vi "_old_Load_SetList_Convert_v2.2_to_v4.vi"(0 "Path":path=path "G:/experiment/Data Acquisition/Hardware Control/procedures/23July07_Evaporate_AO_NoRF_NiceBEC_XY_Opt_Abigail", 1 "error in (no error)":errorcluster) -> (2 "Procedure Name":string="IBS_PICameraTest_29Sep04", 3 "Paramaters":T1={"Master PB Staging List"=[{"Output Bits"=[], "Delay (s)"="", "String"="", "Halt?"=FALSE}, {"Output Bits"=[], "Delay (s)"="", "String"="", "Halt?"=FALSE}, {"Output Bits"=[], "Delay (s)"="", "String"="", "Halt?"=FALSE}, {"Output Bits"=[], "Delay (s)"="", "String"="", "Halt?"=FALSE}, {"Output Bits"=[], "Delay (s)"="", "String"="", "Halt?"=FALSE}, {"Output Bits"=[], "Delay (s)"="", "String"="", "Halt?"=FALSE}, {"Output Bits"=[], "Delay (s)"="", "String"="", "Halt?"=FALSE}, {"Output Bits"=[], "Delay (s)"="", "String"="", "Halt?"=FALSE}, {"Output Bits"=[], "Delay (s)"="", "String"="", "Halt?"=FALSE}, {"Output Bits"=[], "Delay (s)"="", "String"="", "Halt?"=FALSE}, {"Output Bits"=[], "Delay (s)"="", "String"="", "Halt?"=FALSE}, {"Output Bits"=[], "Delay (s)"="", "String"="", "Halt?"=FALSE}, {"Output Bits"=[], "Delay (s)"="", "String"="", "Halt?"=FALSE}, {"Output Bits"=[], "Delay (s)"="", "String"="", "Halt?"=FALSE}, {"Output Bits"=[], "Delay (s)"="", "String"="", "Halt?"=FALSE}, {"Output Bits"=[], "Delay (s)"="", "String"="", "Halt?"=FALSE}, {"Output Bits"=[], "Delay (s)"="", "String"="", "Halt?"=FALSE}, {"Output Bits"=[], "Delay (s)"="", "String"="", "Halt?"=FALSE}, {"Output Bits"=[], "Delay (s)"="", "String"="", "Halt?"=FALSE}, {"Output Bits"=[], "Delay (s)"="", "String"="", "Halt?"=FALSE}, {"Output Bits"=[], "Delay (s)"="", "String"="", "Halt?"=FALSE}, {"Output Bits"=[], "Delay (s)"="", "String"="", "Halt?"=FALSE}, {"Output Bits"=[], "Delay (s)"="", "String"="", "Halt?"=FALSE}, {"Output Bits"=[], "Delay (s)"="", "String"="", "Halt?"=FALSE}, {"Output Bits"=[], "Delay (s)"="", "String"="", "Halt?"=FALSE}, {"Output Bits"=[], "Delay (s)"="", "String"="", "Halt?"=FALSE}, {"Output Bits"=[], "Delay (s)"="", "String"="", "Halt?"=FALSE}, {"Output Bits"=[], "Delay (s)"="", "String"="", "Halt?"=FALSE}, {"Output Bits"=[], "Delay (s)"="", "String"="", "Halt?"=FALSE}, {"Output Bits"=[], "Delay (s)"="", "String"="", "Halt?"=FALSE}, {"Output Bits"=[], "Delay (s)"="", "String"="", "Halt?"=FALSE}, {"Output Bits"=[], "Delay (s)"="", "String"="", "Halt?"=FALSE}, {"Output Bits"=[], "Delay (s)"="", "String"="", "Halt?"=FALSE}, {"Output Bits"=[], "Delay (s)"="", "String"="", "Halt?"=FALSE}, {"Output Bits"=[], "Delay (s)"="", "String"="", "Halt?"=FALSE}, {"Output Bits"=[], "Delay (s)"="", "String"="", "Halt?"=FALSE}, {"Output Bits"=[], "Delay (s)"="", "String"="", "Halt?"=FALSE}, {"Output Bits"=[], "Delay (s)"="", "String"="", "Halt?"=FALSE}, {"Output Bits"=[], "Delay (s)"="", "String"="", "Halt?"=FALSE}, {"Output Bits"=[], "Delay (s)"="", "String"="", "Halt?"=FALSE}, {"Output Bits"=[], "Delay (s)"="", "String"="", "Halt?"=FALSE}, {"Output Bits"=[], "Delay (s)"="", "String"="", "Halt?"=FALSE}, {"Output Bits"=[], "Delay (s)"="", "String"="", "Halt?"=FALSE}, {"Output Bits"=[], "Delay (s)"="", "String"="", "Halt?"=FALSE}], "Slave PB Staging List"=[{"Output Bits"=[], "Delay (s)"="", "String"="", "Halt?"=FALSE}, {"Output Bits"=[], "Delay (s)"="", "String"="", "Halt?"=FALSE}, {"Output Bits"=[], "Delay (s)"="", "String"="", "Halt?"=FALSE}, {"Output Bits"=[], "Delay (s)"="", "String"="", "Halt?"=FALSE}, {"Output Bits"=[], "Delay (s)"="", "String"="", "Halt?"=FALSE}, {"Output Bits"=[], "Delay (s)"="", "String"="", "Halt?"=FALSE}, {"Output Bits"=[], "Delay (s)"="", "String"="", "Halt?"=FALSE}, {"Output Bits"=[], "Delay (s)"="", "String"="", "Halt?"=FALSE}, {"Output Bits"=[], "Delay (s)"="", "String"="", "Halt?"=FALSE}, {"Output Bits"=[], "Delay (s)"="", "String"="", "Halt?"=FALSE}, {"Output Bits"=[], "Delay (s)"="", "String"="", "Halt?"=FALSE}, {"Output Bits"=[], "Delay (s)"="", "String"="", "Halt?"=FALSE}, {"Output Bits"=[], "Delay (s)"="", "String"="", "Halt?"=FALSE}, {"Output Bits"=[], "Delay (s)"="", "String"="", "Halt?"=FALSE}, {"Output Bits"=[], "Delay (s)"="", "String"="", "Halt?"=FALSE}, {"Output Bits"=[], "Delay (s)"="", "String"="", "Halt?"=FALSE}, {"Output Bits"=[], "Delay (s)"="", "String"="", "Halt?"=FALSE}, {"Output Bits"=[], "Delay (s)"="", "String"="", "Halt?"=FALSE}, {"Output Bits"=[], "Delay (s)"="", "String"="", "Halt?"=FALSE}, {"Output Bits"=[], "Delay (s)"="", "String"="", "Halt?"=FALSE}, {"Output Bits"=[], "Delay (s)"="", "String"="", "Halt?"=FALSE}, {"Output Bits"=[], "Delay (s)"="", "String"="", "Halt?"=FALSE}, {"Output Bits"=[], "Delay (s)"="", "String"="", "Halt?"=FALSE}, {"Output Bits"=[], "Delay (s)"="", "String"="", "Halt?"=FALSE}, {"Output Bits"=[], "Delay (s)"="", "String"="", "Halt?"=FALSE}, {"Output Bits"=[], "Delay (s)"="", "String"="", "Halt?"=FALSE}, {"Output Bits"=[], "Delay (s)"="", "String"="", "Halt?"=FALSE}, {"Output Bits"=[], "Delay (s)"="", "String"="", "Halt?"=FALSE}, {"Output Bits"=[], "Delay (s)"="", "String"="", "Halt?"=FALSE}, {"Output Bits"=[], "Delay (s)"="", "String"="", "Halt?"=FALSE}, {"Output Bits"=[], "Delay (s)"="", "String"="", "Halt?"=FALSE}, {"Output Bits"=[], "Delay (s)"="", "String"="", "Halt?"=FALSE}, {"Output Bits"=[], "Delay (s)"="", "String"="", "Halt?"=FALSE}, {"Output Bits"=[], "Delay (s)"="", "String"="", "Halt?"=FALSE}, {"Output Bits"=[], "Delay (s)"="", "String"="", "Halt?"=FALSE}, {"Output Bits"=[], "Delay (s)"="", "String"="", "Halt?"=FALSE}, {"Output Bits"=[], "Delay (s)"="", "String"="", "Halt?"=FALSE}, {"Output Bits"=[], "Delay (s)"="", "String"="", "Halt?"=FALSE}, {"Output Bits"=[], "Delay (s)"="", "String"="", "Halt?"=FALSE}, {"Output Bits"=[], "Delay (s)"="", "String"="", "Halt?"=FALSE}, {"Output Bits"=[], "Delay (s)"="", "String"="", "Halt?"=FALSE}, {"Output Bits"=[], "Delay (s)"="", "String"="", "Halt?"=FALSE}, {"Output Bits"=[], "Delay (s)"="", "String"="", "Halt?"=FALSE}, {"Output Bits"=[], "Delay (s)"="", "String"="", "Halt?"=FALSE}], "Novatech Ramps"=[{"Ramp Channels"=[], "2 Freq. [MHz]"="", "2 Power [dBm]"="", "3 Freq. [MHz]"="", "3 Power [dBm]"="", "Serial Port"=""}, {"Ramp Channels"=[], "2 Freq. [MHz]"="", "2 Power [dBm]"="", "3 Freq. [MHz]"="", "3 Power [dBm]"="", "Serial Port"=""}, {"Ramp Channels"=[], "2 Freq. [MHz]"="", "2 Power [dBm]"="", "3 Freq. [MHz]"="", "3 Power [dBm]"="", "Serial Port"=""}, {"Ramp Channels"=[], "2 Freq. [MHz]"="", "2 Power [dBm]"="", "3 Freq. [MHz]"="", "3 Power [dBm]"="", "Serial Port"=""}, {"Ramp Channels"=[], "2 Freq. [MHz]"="", "2 Power [dBm]"="", "3 Freq. [MHz]"="", "3 Power [dBm]"="", "Serial Port"=""}, {"Ramp Channels"=[], "2 Freq. [MHz]"="", "2 Power [dBm]"="", "3 Freq. [MHz]"="", "3 Power [dBm]"="", "Serial Port"=""}, {"Ramp Channels"=[], "2 Freq. [MHz]"="", "2 Power [dBm]"="", "3 Freq. [MHz]"="", "3 Power [dBm]"="", "Serial Port"=""}], "Sequencing Info"=[{"Start"=0.0, "End"=2.11, "Sequenced Data"=[], "Inform\nIgor?"=FALSE, "Computed Step Size"=0.0, "Procedure Variable"="", "Default"=2.11, "Steps"=0}], "SRS Ramps"=[{"lattice ramp"=[{"dt"="", "formula"=""}, {"dt"="", "formula"=""}, {"dt"="", "formula"=""}], "Output"=[{"Time Values"=[0.0, 0.002, 0.004, 0.006, 0.008, 0.01, 0.012, 0.014, 0.016, 0.018000000000000002, 0.02, 0.022, 0.024, 0.026000000000000002, 0.028, 0.03, 0.032, 0.034, 0.036000000000000004, 0.038, 0.04, 0.042, 0.044, 0.046, 0.048, 0.05, 0.052000000000000005, 0.054, 0.056, 0.058, 0.06, 0.062, 0.064, 0.066, 0.068, 0.07, 0.07200000000000001, 0.074, 0.076, 0.078, 0.08, 0.082, 0.084, 0.08600000000000001, 0.088, 0.09, 0.092, 0.094, 0.096, 0.098, 0.1, 0.10200000000000001, 0.10400000000000001, 0.106, 0.108, 0.11, 0.112, 0.114, 0.116, 0.11800000000000001, 0.12, 0.122, 0.124, 0.126, 0.128, 0.13, 0.132, 0.134, 0.136, 0.138, 0.14, 0.14200000000000002, 0.14400000000000002, 0.146, 0.148, 0.15, 0.152, 0.154, 0.156, 0.158, 0.16, 0.162, 0.164, 0.166, 0.168, 0.17, 0.17200000000000001, 0.17400000000000002, 0.176, 0.178, 0.18, 0.182, 0.184, 0.186, 0.188, 0.19, 0.192, 0.194, 0.196, 0.198, 0.2, 0.6000000000000001, 0.6000000000000001, 0.6002000000000001, 0.6004, 0.6006000000000001, 0.6008000000000001, 0.6010000000000001, 0.6012000000000001, 0.6014, 0.6016000000000001, 0.6018000000000001, 0.6020000000000001, 0.6022000000000001, 0.6024, 0.6026000000000001, 0.6028000000000001, 0.6030000000000001, 0.6032000000000001, 0.6034, 0.6036000000000001, 0.6038000000000001, 0.6040000000000001, 0.6042000000000001, 0.6044, 0.6046000000000001, 0.6048000000000001, 0.6050000000000001, 0.6052000000000001, 0.6054, 0.6056000000000001, 0.6058000000000001, 0.6060000000000001, 0.6062000000000001, 0.6064, 0.6066000000000001, 0.6068000000000001, 0.6070000000000001, 0.6072000000000001, 0.6074, 0.6076000000000001, 0.6078000000000001, 0.6080000000000001, 0.6082000000000001, 0.6084, 0.6086000000000001, 0.6088000000000001, 0.6090000000000001, 0.6092000000000001, 0.6094, 0.6096000000000001, 0.6098000000000001, 0.6100000000000001, 0.6102000000000001, 0.6104, 0.6106000000000001, 0.6108000000000001, 0.6110000000000001, 0.6112000000000001, 0.6114, 0.6116000000000001, 0.6118000000000001, 0.6120000000000001, 0.6122000000000001, 0.6124, 0.6126, 0.6128000000000001, 0.6130000000000001, 0.6132000000000001, 0.6134000000000001, 0.6136000000000001, 0.6138000000000001, 0.6140000000000001, 0.6142000000000001, 0.6144000000000001, 0.6146, 0.6148000000000001, 0.6150000000000001, 0.6152000000000001, 0.6154000000000001, 0.6156, 0.6158000000000001, 0.6160000000000001, 0.6162000000000001, 0.6164000000000001, 0.6166, 0.6168000000000001, 0.6170000000000001, 0.6172000000000001, 0.6174000000000001, 0.6176, 0.6178000000000001, 0.6180000000000001, 0.6182000000000001, 0.6184000000000001, 0.6186, 0.6188000000000001, 0.6190000000000001, 0.6192000000000001, 0.6194000000000001, 0.6196, 0.6198000000000001, 0.6200000000000001, 0.6202000000000001, 0.6212000000000001], array[205 elements]}, {"Time Values"=[0.0, 0.002, 0.004, 0.006, 0.008, 0.01, 0.012, 0.014, 0.016, 0.018000000000000002, 0.02, 0.022, 0.024, 0.026000000000000002, 0.028, 0.03, 0.032, 0.034, 0.036000000000000004, 0.038, 0.04, 0.042, 0.044, 0.046, 0.048, 0.05, 0.052000000000000005, 0.054, 0.056, 0.058, 0.06, 0.062, 0.064, 0.066, 0.068, 0.07, 0.07200000000000001, 0.074, 0.076, 0.078, 0.08, 0.082, 0.084, 0.08600000000000001, 0.088, 0.09, 0.092, 0.094, 0.096, 0.098, 0.1, 0.10200000000000001, 0.10400000000000001, 0.106, 0.108, 0.11, 0.112, 0.114, 0.116, 0.11800000000000001, 0.12, 0.122, 0.124, 0.126, 0.128, 0.13, 0.132, 0.134, 0.136, 0.138, 0.14, 0.14200000000000002, 0.14400000000000002, 0.146, 0.148, 0.15, 0.152, 0.154, 0.156, 0.158, 0.16, 0.162, 0.164, 0.166, 0.168, 0.17, 0.17200000000000001, 0.17400000000000002, 0.176, 0.178, 0.18, 0.182, 0.184, 0.186, 0.188, 0.19, 0.192, 0.194, 0.196, 0.198, 0.2, 0.6000000000000001, 0.6000000000000001, 0.6002000000000001, 0.6004, 0.6006000000000001, 0.6008000000000001, 0.6010000000000001, 0.6012000000000001, 0.6014, 0.6016000000000001, 0.6018000000000001, 0.6020000000000001, 0.6022000000000001, 0.6024, 0.6026000000000001, 0.6028000000000001, 0.6030000000000001, 0.6032000000000001, 0.6034, 0.6036000000000001, 0.6038000000000001, 0.6040000000000001, 0.6042000000000001, 0.6044, 0.6046000000000001, 0.6048000000000001, 0.6050000000000001, 0.6052000000000001, 0.6054, 0.6056000000000001, 0.6058000000000001, 0.6060000000000001, 0.6062000000000001, 0.6064, 0.6066000000000001, 0.6068000000000001, 0.6070000000000001, 0.6072000000000001, 0.6074, 0.6076000000000001, 0.6078000000000001, 0.6080000000000001, 0.6082000000000001, 0.6084, 0.6086000000000001, 0.6088000000000001, 0.6090000000000001, 0.6092000000000001, 0.6094, 0.6096000000000001, 0.6098000000000001, 0.6100000000000001, 0.6102000000000001, 0.6104, 0.6106000000000001, 0.6108000000000001, 0.6110000000000001, 0.6112000000000001, 0.6114, 0.6116000000000001, 0.6118000000000001, 0.6120000000000001, 0.6122000000000001, 0.6124, 0.6126, 0.6128000000000001, 0.6130000000000001, 0.6132000000000001, 0.6134000000000001, 0.6136000000000001, 0.6138000000000001, 0.6140000000000001, 0.6142000000000001, 0.6144000000000001, 0.6146, 0.6148000000000001, 0.6150000000000001, 0.6152000000000001, 0.6154000000000001, 0.6156, 0.6158000000000001, 0.6160000000000001, 0.6162000000000001, 0.6164000000000001, 0.6166, 0.6168000000000001, 0.6170000000000001, 0.6172000000000001, 0.6174000000000001, 0.6176, 0.6178000000000001, 0.6180000000000001, 0.6182000000000001, 0.6184000000000001, 0.6186, 0.6188000000000001, 0.6190000000000001, 0.6192000000000001, 0.6194000000000001, 0.6196, 0.6198000000000001, 0.6200000000000001, 0.6202000000000001, 0.6212000000000001], array[205 elements]}], "SRS Selection"=enum."1550 Vertical"}, {"lattice ramp"=[{"dt"="", "formula"=""}], "Output"=[{"Time Values"=[0.0, 0.002, 0.004, 0.006, 0.008, 0.01, 0.012, 0.014, 0.016, 0.018000000000000002, 0.02, 0.022, 0.024, 0.026000000000000002, 0.028, 0.03, 0.032, 0.034, 0.036000000000000004, 0.038, 0.04, 0.042, 0.044, 0.046, 0.048, 0.05, 0.052000000000000005, 0.054, 0.056, 0.058, 0.06, 0.062, 0.064, 0.066, 0.068, 0.07, 0.07200000000000001, 0.074, 0.076, 0.078, 0.08, 0.082, 0.084, 0.08600000000000001, 0.088, 0.09, 0.092, 0.094, 0.096, 0.098, 0.1, 0.10200000000000001, 0.10400000000000001, 0.106, 0.108, 0.11, 0.112, 0.114, 0.116, 0.11800000000000001, 0.12, 0.122, 0.124, 0.126, 0.128, 0.13, 0.132, 0.134, 0.136, 0.138, 0.14, 0.14200000000000002, 0.14400000000000002, 0.146, 0.148, 0.15, 0.152, 0.154, 0.156, 0.158, 0.16, 0.162, 0.164, 0.166, 0.168, 0.17, 0.17200000000000001, 0.17400000000000002, 0.176, 0.178, 0.18, 0.182, 0.184, 0.186, 0.188, 0.19, 0.192, 0.194, 0.196, 0.198, 0.2, 0.6000000000000001, 0.6000000000000001, 0.6002000000000001, 0.6004, 0.6006000000000001, 0.6008000000000001, 0.6010000000000001, 0.6012000000000001, 0.6014, 0.6016000000000001, 0.6018000000000001, 0.6020000000000001, 0.6022000000000001, 0.6024, 0.6026000000000001, 0.6028000000000001, 0.6030000000000001, 0.6032000000000001, 0.6034, 0.6036000000000001, 0.6038000000000001, 0.6040000000000001, 0.6042000000000001, 0.6044, 0.6046000000000001, 0.6048000000000001, 0.6050000000000001, 0.6052000000000001, 0.6054, 0.6056000000000001, 0.6058000000000001, 0.6060000000000001, 0.6062000000000001, 0.6064, 0.6066000000000001, 0.6068000000000001, 0.6070000000000001, 0.6072000000000001, 0.6074, 0.6076000000000001, 0.6078000000000001, 0.6080000000000001, 0.6082000000000001, 0.6084, 0.6086000000000001, 0.6088000000000001, 0.6090000000000001, 0.6092000000000001, 0.6094, 0.6096000000000001, 0.6098000000000001, 0.6100000000000001, 0.6102000000000001, 0.6104, 0.6106000000000001, 0.6108000000000001, 0.6110000000000001, 0.6112000000000001, 0.6114, 0.6116000000000001, 0.6118000000000001, 0.6120000000000001, 0.6122000000000001, 0.6124, 0.6126, 0.6128000000000001, 0.6130000000000001, 0.6132000000000001, 0.6134000000000001, 0.6136000000000001, 0.6138000000000001, 0.6140000000000001, 0.6142000000000001, 0.6144000000000001, 0.6146, 0.6148000000000001, 0.6150000000000001, 0.6152000000000001, 0.6154000000000001, 0.6156, 0.6158000000000001, 0.6160000000000001, 0.6162000000000001, 0.6164000000000001, 0.6166, 0.6168000000000001, 0.6170000000000001, 0.6172000000000001, 0.6174000000000001, 0.6176, 0.6178000000000001, 0.6180000000000001, 0.6182000000000001, 0.6184000000000001, 0.6186, 0.6188000000000001, 0.6190000000000001, 0.6192000000000001, 0.6194000000000001, 0.6196, 0.6198000000000001, 0.6200000000000001, 0.6202000000000001, 0.6212000000000001], array[205 elements]}, {"Time Values"=[0.0, 0.002, 0.004, 0.006, 0.008, 0.01, 0.012, 0.014, 0.016, 0.018000000000000002, 0.02, 0.022, 0.024, 0.026000000000000002, 0.028, 0.03, 0.032, 0.034, 0.036000000000000004, 0.038, 0.04, 0.042, 0.044, 0.046, 0.048, 0.05, 0.052000000000000005, 0.054, 0.056, 0.058, 0.06, 0.062, 0.064, 0.066, 0.068, 0.07, 0.07200000000000001, 0.074, 0.076, 0.078, 0.08, 0.082, 0.084, 0.08600000000000001, 0.088, 0.09, 0.092, 0.094, 0.096, 0.098, 0.1, 0.10200000000000001, 0.10400000000000001, 0.106, 0.108, 0.11, 0.112, 0.114, 0.116, 0.11800000000000001, 0.12, 0.122, 0.124, 0.126, 0.128, 0.13, 0.132, 0.134, 0.136, 0.138, 0.14, 0.14200000000000002, 0.14400000000000002, 0.146, 0.148, 0.15, 0.152, 0.154, 0.156, 0.158, 0.16, 0.162, 0.164, 0.166, 0.168, 0.17, 0.17200000000000001, 0.17400000000000002, 0.176, 0.178, 0.18, 0.182, 0.184, 0.186, 0.188, 0.19, 0.192, 0.194, 0.196, 0.198, 0.2, 0.6000000000000001, 0.6000000000000001, 0.6002000000000001, 0.6004, 0.6006000000000001, 0.6008000000000001, 0.6010000000000001, 0.6012000000000001, 0.6014, 0.6016000000000001, 0.6018000000000001, 0.6020000000000001, 0.6022000000000001, 0.6024, 0.6026000000000001, 0.6028000000000001, 0.6030000000000001, 0.6032000000000001, 0.6034, 0.6036000000000001, 0.6038000000000001, 0.6040000000000001, 0.6042000000000001, 0.6044, 0.6046000000000001, 0.6048000000000001, 0.6050000000000001, 0.6052000000000001, 0.6054, 0.6056000000000001, 0.6058000000000001, 0.6060000000000001, 0.6062000000000001, 0.6064, 0.6066000000000001, 0.6068000000000001, 0.6070000000000001, 0.6072000000000001, 0.6074, 0.6076000000000001, 0.6078000000000001, 0.6080000000000001, 0.6082000000000001, 0.6084, 0.6086000000000001, 0.6088000000000001, 0.6090000000000001, 0.6092000000000001, 0.6094, 0.6096000000000001, 0.6098000000000001, 0.6100000000000001, 0.6102000000000001, 0.6104, 0.6106000000000001, 0.6108000000000001, 0.6110000000000001, 0.6112000000000001, 0.6114, 0.6116000000000001, 0.6118000000000001, 0.6120000000000001, 0.6122000000000001, 0.6124, 0.6126, 0.6128000000000001, 0.6130000000000001, 0.6132000000000001, 0.6134000000000001, 0.6136000000000001, 0.6138000000000001, 0.6140000000000001, 0.6142000000000001, 0.6144000000000001, 0.6146, 0.6148000000000001, 0.6150000000000001, 0.6152000000000001, 0.6154000000000001, 0.6156, 0.6158000000000001, 0.6160000000000001, 0.6162000000000001, 0.6164000000000001, 0.6166, 0.6168000000000001, 0.6170000000000001, 0.6172000000000001, 0.6174000000000001, 0.6176, 0.6178000000000001, 0.6180000000000001, 0.6182000000000001, 0.6184000000000001, 0.6186, 0.6188000000000001, 0.6190000000000001, 0.6192000000000001, 0.6194000000000001, 0.6196, 0.6198000000000001, 0.6200000000000001, 0.6202000000000001, 0.6212000000000001], array[205 elements]}], "SRS Selection"=enum."1550 Vertical"}], "Master AO Ramp List"=[{"Ramp index"=10, "Ramp time [s]"="", "Step size [s]"=1000.0, "Ramp Array"=[], "Output Bits"=[]}, {"Ramp index"=10, "Ramp time [s]"="", "Step size [s]"=1000.0, "Ramp Array"=[], "Output Bits"=[]}], "Slave AO Ramp List"=[{"Ramp index"=10, "Ramp time [s]"="", "Step size [s]"=1000.0, "Ramp Array"=[], "Output Bits"=[]}, {"Ramp index"=10, "Ramp time [s]"="", "Step size [s]"=1000.0, "Ramp Array"=[], "Output Bits"=[]}], "Master Novatech Ramp List"=[], "Static Variables"=[], "DDS Ramp List"=[]} {"Static Variables"."Value" format="%#_7p"; "Sequencing Info"."Steps" min=2; "Sequencing Info"."Default" format="%#.7p"; "Sequencing Info"."Computed Step Size" format="%#.7p"; "Sequencing Info"."Sequenced Data" format="%.2e"; "Sequencing Info"."End" format="%#.7p"; "Sequencing Info"."Start" format="%#.7p"}, 4 "error out":errorcluster)   [LabVIEW 2013]
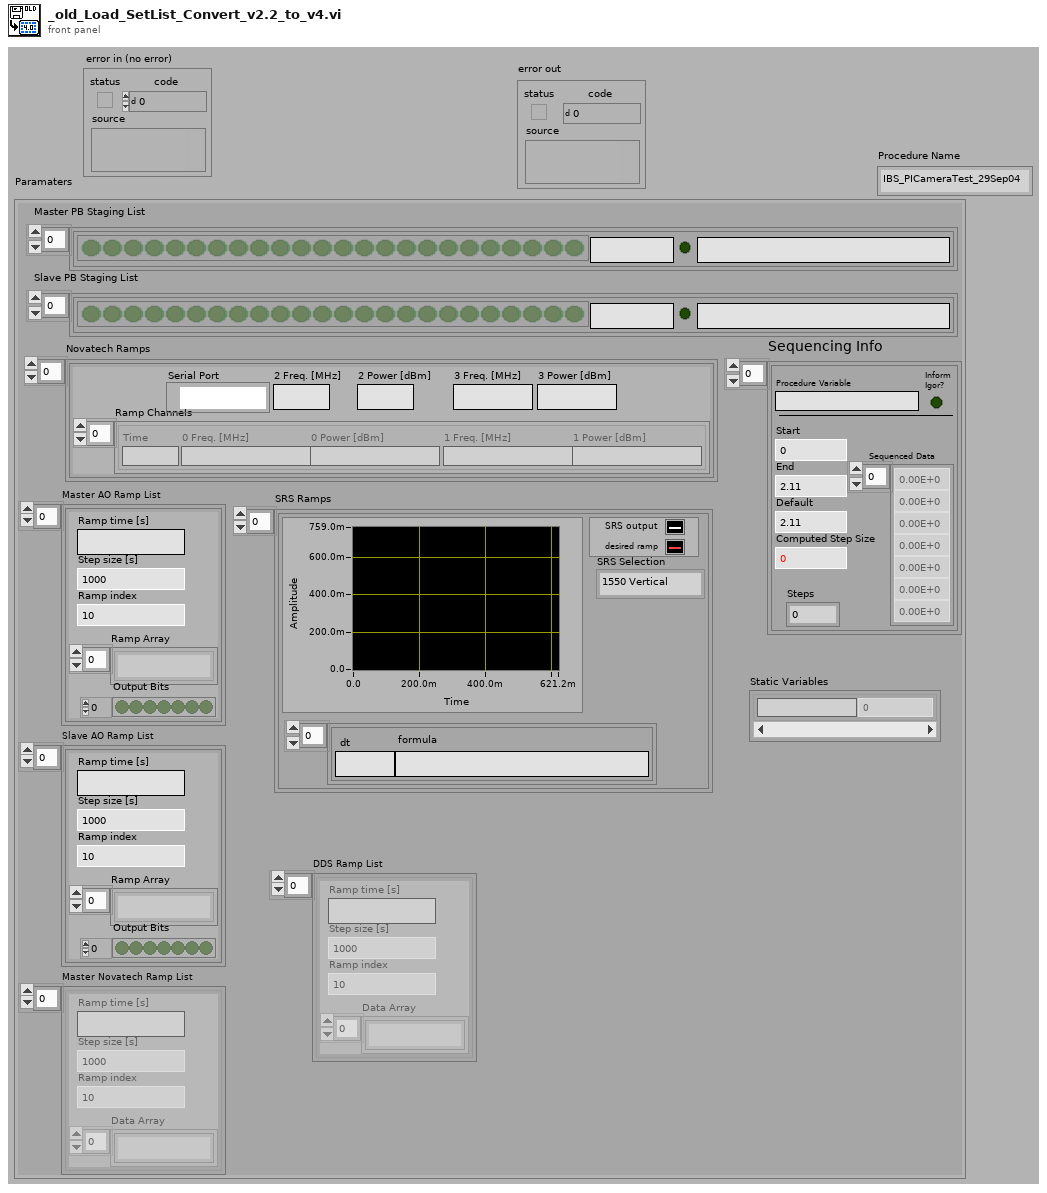
[diagram p1: front panel]
types:
  T1 = cluster{"Master PB Staging List":cluster{"Output Bits":bool[], "Delay (s)":string, "String":string, "Halt?":bool}[], "Slave PB Staging List":cluster{"Output Bits":bool[], "Delay (s)":string, "String":string, "Halt?":bool}[], "Novatech Ramps":cluster{"Ramp Channels":cluster{"Time":string, "0 Freq. [MHz]":string, "0 Power [dBm]":string, "1 Freq. [MHz]":string, "1 Power [dBm]":string}[], "2 Freq. [MHz]":string, "2 Power [dBm]":string, "3 Freq. [MHz]":string, "3 Power [dBm]":string, "Serial Port":refnum<visa-resource-name>}[], "Sequencing Info":cluster{"Start":dbl, "End":dbl, "Sequenced Data":dbl[], "Inform\nIgor?":bool, "Computed Step Size":dbl, "Procedure Variable":string, "Default":dbl, "Steps":i32}[], "SRS Ramps":cluster{"lattice ramp":cluster{"dt":string, "formula":string}[], "Output":cluster{"Time Values":dbl[], dbl[]}[], "SRS Selection":enum16{"1550 Vertical", "Bragg Agilent", "Bragg PTS", "Acc. Intensity"}}[], "Master AO Ramp List":cluster{"Ramp index":u32, "Ramp time [s]":string, "Step size [s]":dbl, "Ramp Array":string[], "Output Bits":bool[]}[], "Slave AO Ramp List":cluster{"Ramp index":u32, "Ramp time [s]":string, "Step size [s]":dbl, "Ramp Array":string[], "Output Bits":bool[]}[], "Master Novatech Ramp List":cluster{"Ramp index":u32, "Ramp time [s]":string, "Step size [s]":dbl, "Data Array":string[]}[], "Static Variables":cluster{"Procedure variable":string, "Value":dbl}[], "DDS Ramp List":cluster{"Ramp index":u32, "Ramp time [s]":string, "Step size [s]":dbl, "Data Array":string[]}[]}
  T2 = cluster{"Ramp index":u32, "Ramp time [s]":string, "Step size [s]":dbl, "Data Array":string[]}[]
  T3 = cluster{"Master PB Staging List":cluster{"Output Bits":bool[], "Delay (s)":dbl, "String":string, "Halt?":bool}[], "Slave PB Staging List":cluster{"Output Bits":bool[], "Delay (s)":dbl, "String":string, "Halt?":bool}[], "Master AO Staging List":dbl[][], "Slave AO Staging List":dbl[][], "Master AO Ramp List":cluster{"Ramp time":dbl, "Nsteps":u32, "Ramp index":u32, "Start Values":dbl[], "Stop Values":dbl[], "Ramp\nType":enum16{"none", "AO", "AI"}}[], "Slave AO Ramp List":cluster{"Ramp time":dbl, "Nsteps":u32, "Ramp index":u32, "Start Values":dbl[], "Stop Values":dbl[], "Ramp\nType":enum16{"none", "AO", "AI"}}[], "Evaporation Params":cluster{"RF Sweep ?":bool, "RF ramp list":cluster{"Time":dbl, "Frequency [MHz]":dbl, "Power [dBm]":dbl}[]}, "Sequencing Info":cluster{"Start":dbl, "End":dbl, "Sequenced Data":dbl[], "Sequence Data Source":bool, "Scan Staging List":enum16{"Master", "Slave"}, "Index to Scan":i16, "Scan Type":enum16{"PB delay", "AO", "Evap Time", "Evap Amp", "Evap Freq", "Agilent fixed waveform", "Agilent sweep", "Variable Ramp"}, "AO/ RT Channel":i16, "Igor Inform variable":string, "Inform?":bool, "Computed Step Size":dbl, "SRS/RT Line":i16}[], "SRS Ramps":cluster{"lattice ramp":cluster{"a":dbl, "dt":dbl, "Ramp Type":enum16{"Hold=a", "Lin (a to b)", "Exp, (a to b with tau=c)", "Sin=a+b*sin(2*pi*c*t)", "SG a=off, c=f, b=amp", "Blackman (a = amp)", "HGauss (a to b, width c)", "Chirp (a+b*sin(2*pi*f*t)), f from c to d"}, "b":dbl, "c":dbl}[], "Output":cluster{"Time Values":dbl[], dbl[]}[], "SRS Selection":enum16{"1550 Vertical", "Bragg Agilent", "Bragg PTS", "Acc. Intensity"}}[], "Agilent built-in fxns array":cluster{"Agilent sweep parameters":cluster{"Lower Frequency [Hz][0]":dbl, "Upper Frequency [Hz][1]":dbl, "Sweep Mode (0: Off)":u16, "Sweep Spacing (0: Linear up)":u16, "Sweep Time [s]":dbl}, "Agilent fixed waveform parameters":cluster{"Frequency [Hz]":dbl, "Offset [V]":dbl, "Waveform Shape":u16, "Amplitude [Vpp]":dbl}, "Agilent selection":u16, "Function selection":u16, "Agilent phase shift parameter":cluster{"Phase [deg]":dbl, "FSK pulse length [s]":dbl}, "Ring":u16}[]}
  T4 = cluster{"Output Bits":bool[], "Delay (s)":dbl, "String":string, "Halt?":bool}[]
  T5 = cluster{"Ramp time":dbl, "Nsteps":u32, "Ramp index":u32, "Start Values":dbl[], "Stop Values":dbl[], "Ramp\nType":enum16{"none", "AO", "AI"}}[]
  T6 = cluster{"RF Sweep ?":bool, "RF ramp list":cluster{"Time":dbl, "Frequency [MHz]":dbl, "Power [dBm]":dbl}[]}
  T7 = cluster{"Start":dbl, "End":dbl, "Sequenced Data":dbl[], "Sequence Data Source":bool, "Scan Staging List":enum16{"Master", "Slave"}, "Index to Scan":i16, "Scan Type":enum16{"PB delay", "AO", "Evap Time", "Evap Amp", "Evap Freq", "Agilent fixed waveform", "Agilent sweep", "Variable Ramp"}, "AO/ RT Channel":i16, "Igor Inform variable":string, "Inform?":bool, "Computed Step Size":dbl, "SRS/RT Line":i16}[]
  T8 = cluster{"lattice ramp":cluster{"a":dbl, "dt":dbl, "Ramp Type":enum16{"Hold=a", "Lin (a to b)", "Exp, (a to b with tau=c)", "Sin=a+b*sin(2*pi*c*t)", "SG a=off, c=f, b=amp", "Blackman (a = amp)", "HGauss (a to b, width c)", "Chirp (a+b*sin(2*pi*f*t)), f from c to d"}, "b":dbl, "c":dbl}[], "Output":cluster{"Time Values":dbl[], dbl[]}[], "SRS Selection":enum16{"1550 Vertical", "Bragg Agilent", "Bragg PTS", "Acc. Intensity"}}[]
  T9 = cluster{"Output Bits":bool[], "Delay (s)":string, "String":string, "Halt?":bool}[]
  T10 = cluster{"Output Bits":bool[], "Delay (s)":string, "String":string, "Halt?":bool}
  T11 = cluster{"Start":dbl, "End":dbl, "Sequenced Data":dbl[], "Inform\nIgor?":bool, "Computed Step Size":dbl, "Procedure Variable":string, "Default":dbl, "Steps":i32}[]
  T12 = cluster{"Start":dbl, "End":dbl, "Sequenced Data":dbl[], "Inform\nIgor?":bool, "Computed Step Size":dbl, "Procedure Variable":string, "Default":dbl, "Steps":i32}
  T13 = cluster{"Time":dbl, "Frequency [MHz]":dbl, "Power [dBm]":dbl}[]
  T14 = cluster{"Ramp Channels":cluster{"Time":string, "0 Freq. [MHz]":string, "0 Power [dBm]":string, "1 Freq. [MHz]":string, "1 Power [dBm]":string}[], "2 Freq. [MHz]":string, "2 Power [dBm]":string, "3 Freq. [MHz]":string, "3 Power [dBm]":string, "Serial Port":refnum<visa-resource-name>}[]
  T15 = cluster{"Ramp Channels":cluster{"Time":string, "0 Freq. [MHz]":string, "0 Power [dBm]":string, "1 Freq. [MHz]":string, "1 Power [dBm]":string}[], "2 Freq. [MHz]":string, "2 Power [dBm]":string, "3 Freq. [MHz]":string, "3 Power [dBm]":string, "Serial Port":refnum<visa-resource-name>}
  T16 = cluster{"Time":string, "0 Freq. [MHz]":string, "0 Power [dBm]":string, "1 Freq. [MHz]":string, "1 Power [dBm]":string}[]
  T17 = cluster{"Time":string, "0 Freq. [MHz]":string, "0 Power [dBm]":string, "1 Freq. [MHz]":string, "1 Power [dBm]":string}
  T18 = cluster{"Time":dbl, "Frequency [MHz]":dbl, "Power [dBm]":dbl}
  T19 = cluster{"lattice ramp":cluster{"dt":string, "formula":string}[], "Output":cluster{"Time Values":dbl[], dbl[]}[], "SRS Selection":enum16{"1550 Vertical", "Bragg Agilent", "Bragg PTS", "Acc. Intensity"}}[]
  T20 = cluster{"lattice ramp":cluster{"dt":string, "formula":string}[], "Output":cluster{"Time Values":dbl[], dbl[]}[], "SRS Selection":enum16{"1550 Vertical", "Bragg Agilent", "Bragg PTS", "Acc. Intensity"}}
  T21 = enum16{"1550 Vertical", "Bragg Agilent", "Bragg PTS", "Acc. Intensity"}
  T22 = cluster{"a":dbl, "dt":dbl, "Ramp Type":enum16{"Hold=a", "Lin (a to b)", "Exp, (a to b with tau=c)", "Sin=a+b*sin(2*pi*c*t)", "SG a=off, c=f, b=amp", "Blackman (a = amp)", "HGauss (a to b, width c)", "Chirp (a+b*sin(2*pi*f*t)), f from c to d"}, "b":dbl, "c":dbl}[]
  T23 = enum16{"Hold=a", "Lin (a to b)", "Exp, (a to b with tau=c)", "Sin=a+b*sin(2*pi*c*t)", "SG a=off, c=f, b=amp", "Blackman (a = amp)", "HGauss (a to b, width c)", "Chirp (a+b*sin(2*pi*f*t)), f from c to d"}
  T24 = cluster{"Ramp index":u32, "Ramp time [s]":string, "Step size [s]":dbl, "Ramp Array":string[], "Output Bits":bool[]}[]
  T25 = cluster{"Ramp index":u32, "Ramp time [s]":string, "Step size [s]":dbl, "Ramp Array":string[], "Output Bits":bool[]}
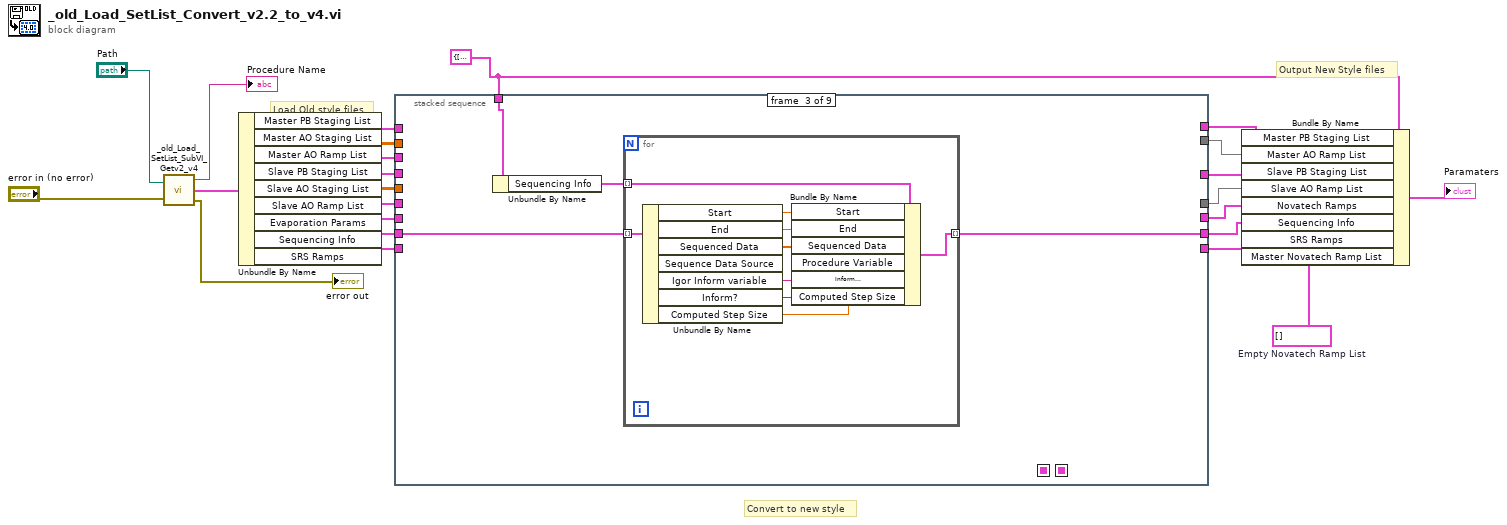
[diagram p0: block diagram]
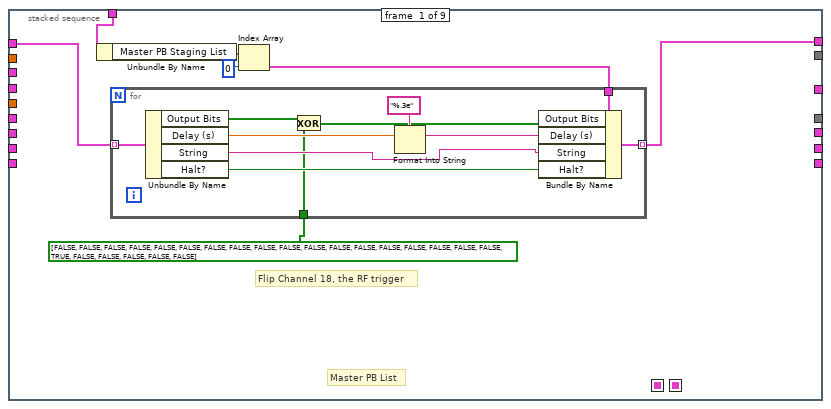
[diagram p2: hidden frame]
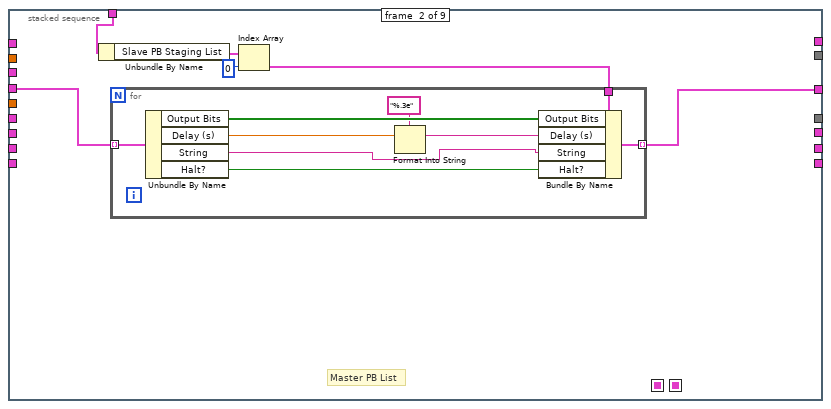
[diagram p3: hidden frame]
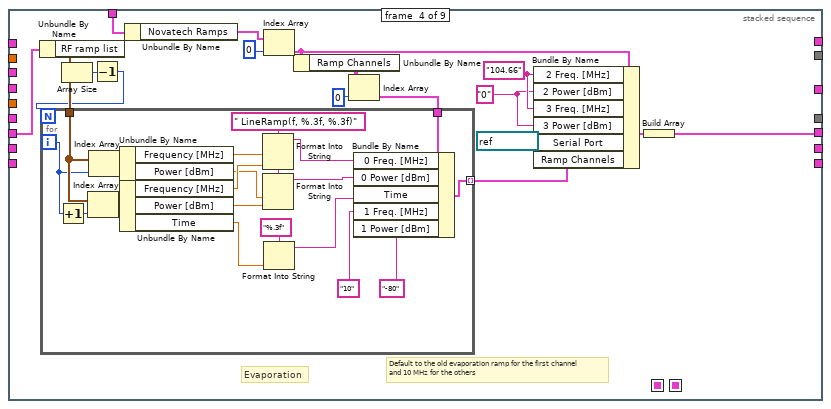
[diagram p4: hidden frame]
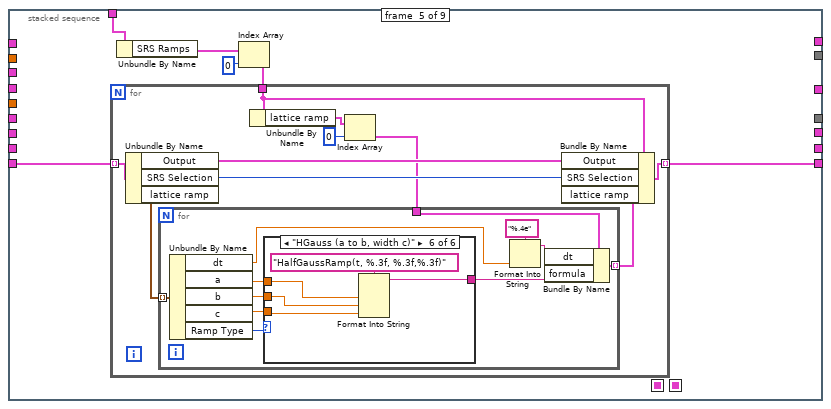
[diagram p5: hidden frame]
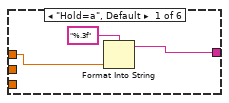
[diagram p6: hidden frame]
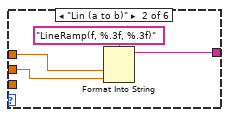
[diagram p7: hidden frame]
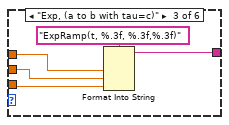
[diagram p8: hidden frame]
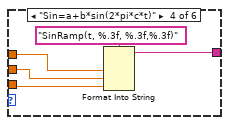
[diagram p9: hidden frame]
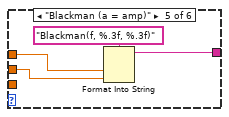
[diagram p10: hidden frame]
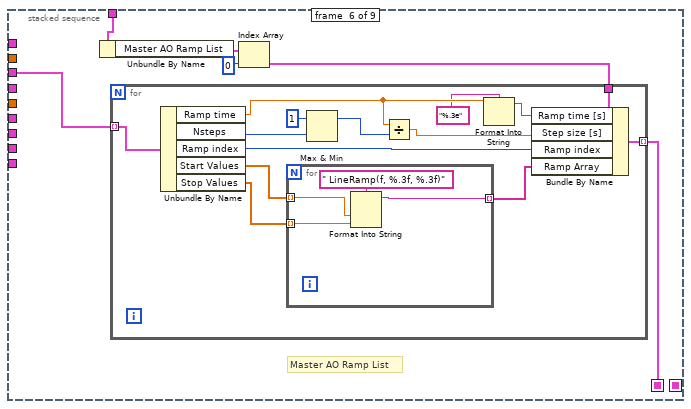
[diagram p11: hidden frame]
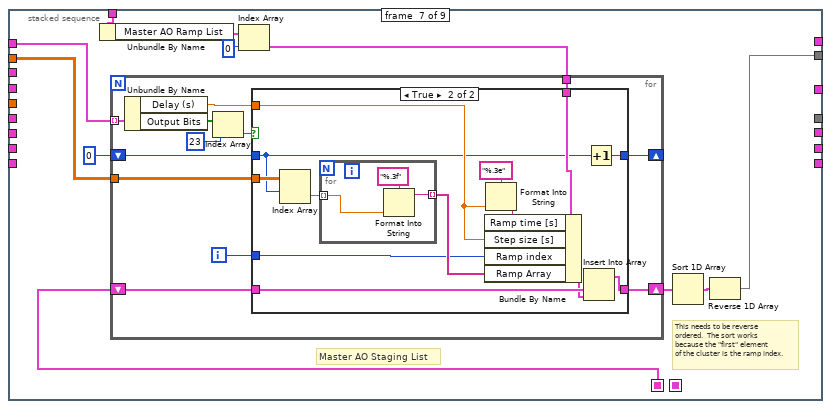
[diagram p12: hidden frame]
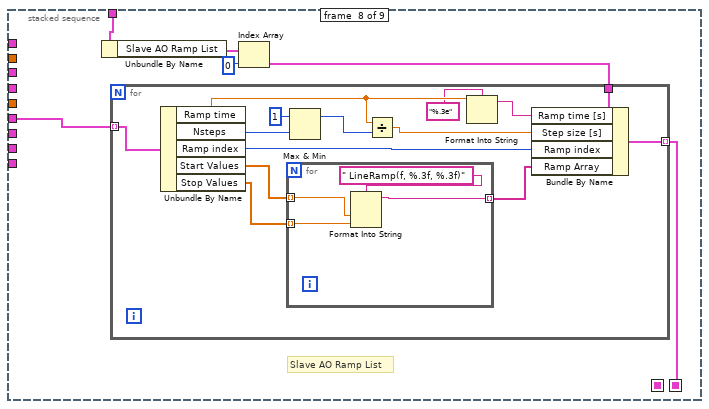
[diagram p14: hidden frame]
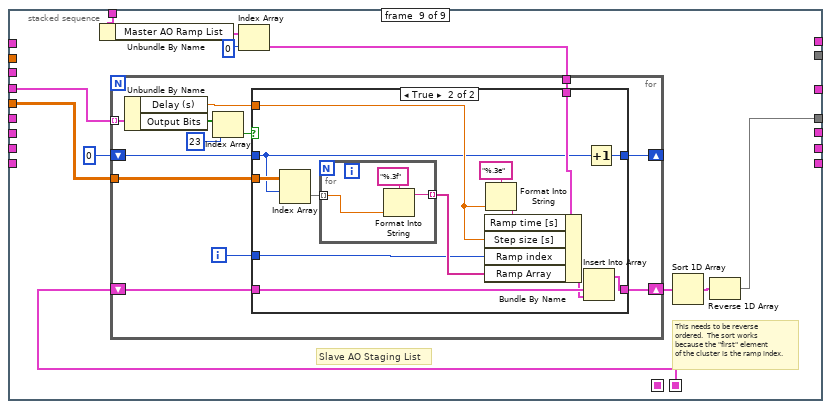
[diagram p15: hidden frame]
diagram:
  w1 = T1 {"Master PB Staging List"=[], "Slave PB Staging List"=[], "Novatech Ramps"=[], "Sequencing Info"=[], "SRS Ramps"=[], "Master AO Ramp List"=[], "Slave AO Ramp List"=[], "Master Novatech Ramp List"=[], "Static Variables"=[], "DDS Ramp List"=[]} ("Paramaters")
  w2 = T2 []  # Empty Novatech Ramp List
  # "Output New Style files"
  # "Convert to new style"
  # "Load Old style files"
  n1 = call "_old_Load_SetList_SubVI_Getv2_v4.vi"("Path"="Path", "error in (no error)"="error in (no error)") -> ("Procedure Name"=→"Procedure Name":string, "Paramaters"=w23:T3, "error out"=→"error out":errorcluster)
  n2 = Unbundle By Name(w23) -> ("Master PB Staging List"=w22:T4, "Master AO Staging List"=w21:dbl[][], "Master AO Ramp List"=w20:T5, "Slave PB Staging List"=w19:T4, "Slave AO Staging List"=w18:dbl[][], "Slave AO Ramp List"=w17:T5, "Evaporation Params"=w16:T6, "Sequencing Info"=w15:T7, "SRS Ramps"=w14:T8)
  n3 = stacked-sequence {
    seq-local: [_ _ _ _ _ w160 _ _ _] -> [_ _ _ _ _ _ w189 _ _]
    seq-local: [_ _ _ _ _ _ _ w225 _] -> [_ _ _ _ _ _ _ _ w249]
    tunnel: w22 -> [w27 _ _ _ _ _ w190 _ _]
    tunnel: w21 -> [_ _ _ _ _ _ w187 _ _]
    tunnel: w20 -> [_ _ _ _ _ w161 _ _ _]
    tunnel: w19 -> [_ w44 _ _ _ _ _ _ w250]
    tunnel: w18 -> [_ _ _ _ _ _ _ _ w251]
    tunnel: w17 -> [_ _ _ _ _ _ _ w226 _]
    tunnel: w16 -> [_ _ _ w87 _ _ _ _ _]
    tunnel: w15 -> [_ _ w61 _ _ _ _ _ _]
    tunnel: w14 -> [_ _ _ _ w111 _ _ _ _]
    tunnel: [w26 _ _ _ _ _ _ _ _] -> w13
    tunnel: [_ w43 _ _ _ _ _ _ _] -> w12
    tunnel: [_ _ w60 _ _ _ _ _ _] -> w11
    tunnel: [_ _ _ w80 _ _ _ _ _] -> w7
    tunnel: w1 -> [w28 w45 w59 w86 w112 w165 w194 w230 w259]
    tunnel: [_ _ _ _ w107 _ _ _ _] -> w10
    tunnel: [_ _ _ _ _ _ w184 _ _] -> w9
    tunnel: [_ _ _ _ _ _ _ _ w252] -> w8
    frame #0 {
      # "Flip Channel 18, the RF trigger"
      # "Master PB List"
      n4 = Unbundle By Name(w28) -> ("Master PB Staging List"=w29:T9)
      n5 = Index Array(array=w29, index=0) -> (element=w31:T10)
      n6 = for {
        tunnel: w31 -> [w42]
        tunnel: w27 -> [w40] mode=indexing
        tunnel: [w41] -> w26 mode=indexing
        tunnel: bool[] [FALSE, FALSE, FALSE, FALSE, FALSE, FALSE, FALSE, FALSE, FALSE, FALSE, FALSE, FALSE, FALSE, FALSE, FALSE, FALSE, FALSE, FALSE, TRUE, FALSE, FALSE, FALSE, FALSE, FALSE] ("Output Bits") -> [w32]
        n7 = Unbundle By Name(w40) -> ("Output Bits"=w34:bool[], "Delay (s)"=w38:dbl, "String"=w36:string, "Halt?"=w35:bool)
        n8 = Exclusive Or(1:w32, 2:w34) -> (0:w33:bool[])
        n9 = Format Into String(format string="%.3e", w38) -> (resulting string=w39:string)  [unwired: 2 in, 1 out]
        n10 = Bundle By Name(cluster=w42, "Output Bits"=w33, "Delay (s)"=w39, "String"=w36, "Halt?"=w35) -> (w41:T10)
      }
    }
    frame #1 {
      # "Master PB List"
      n11 = Unbundle By Name(w45) -> ("Slave PB Staging List"=w46:T9)
      n12 = Index Array(array=w46, index=0) -> (element=w48:T10)
      n13 = for {
        tunnel: w48 -> [w57]
        tunnel: w44 -> [w55] mode=indexing
        tunnel: [w56] -> w43 mode=indexing
        n14 = Unbundle By Name(w55) -> ("Output Bits"=w54:bool[], "Delay (s)"=w52:dbl, "String"=w50:string, "Halt?"=w49:bool)
        n15 = Format Into String(format string="%.3e", w52) -> (resulting string=w53:string)  [unwired: 2 in, 1 out]
        n16 = Bundle By Name(cluster=w57, "Output Bits"=w54, "Delay (s)"=w53, "String"=w50, "Halt?"=w49) -> (w56:T10)
      }
    }
    frame #2 {
      n17 = Unbundle By Name(w59) -> ("Sequencing Info"=w58:T11)
      n18 = for {
        tunnel: w61 -> [w69] mode=indexing
        tunnel: [w62] -> w60 mode=indexing
        tunnel: w58 -> [w70] mode=indexing
        n19 = Unbundle By Name(w69) -> ("Start"=w68:dbl, "End"=w67:dbl, "Sequenced Data"=w66:dbl[], "Igor Inform variable"=w65:string, "Inform?"=w64:bool, "Computed Step Size"=w63:dbl)  [unwired: 1 out]
        n20 = Bundle By Name(cluster=w70, "Start"=w68, "End"=w67, "Sequenced Data"=w66, "Procedure Variable"=w65, "Inform\nIgor?"=w64, "Computed Step Size"=w63) -> (w62:T12)
      }
    }
    frame #3 {
      w77 = "0"
      w78 = "104.66"
      # "Default to the old evaporation ramp for the first channel\nand 10 MHz for the others"
      # "Evaporation"
      n21 = Unbundle By Name(w87) -> ("RF ramp list"=w72:T13)
      n22 = Array Size(array=w72) -> (size(s)=w73:i32)
      n23 = Decrement(x=w73) -> (x-1=w71:i32)
      n24 = Unbundle By Name(w86) -> ("Novatech Ramps"=w84:T14)
      n25 = Index Array(array=w84, index=0) -> (element=w83:T15)
      n26 = Unbundle By Name(w83) -> ("Ramp Channels"=w75:T16)
      n27 = Index Array(array=w75, index=0) -> (element=w74:T17)
      n28 = for {
        N: w71 -> [_]
        tunnel: w72 -> [w102]
        tunnel: [w104] -> w82 mode=indexing
        tunnel: w74 -> [w103]
        i -> [w100]
        w92 = " LineRamp(f, %.3f, %.3f)"
        n29 = Increment(x=w100) -> (x+1=w101:i32)
        n30 = Index Array(array=w102, index=w101) -> (element=w99:T18)
        n31 = Index Array(array=w102, index=w100) -> (element=w98:T18)
        n32 = Unbundle By Name(w98) -> ("Frequency [MHz]"=w91:dbl, "Power [dBm]"=w89:dbl)
        n33 = Unbundle By Name(w99) -> ("Frequency [MHz]"=w90:dbl, "Power [dBm]"=w88:dbl, "Time"=w106:dbl)
        n34 = Format Into String(format string=w92, w91, w90) -> (resulting string=w94:string)  [unwired: 2 in, 1 out]
        n35 = Format Into String(format string=w92, w89, w88) -> (resulting string=w93:string)  [unwired: 2 in, 1 out]
        n36 = Format Into String(format string="%.3f", w106) -> (resulting string=w95:string)  [unwired: 2 in, 1 out]
        n37 = Bundle By Name(cluster=w103, "0 Freq. [MHz]"=w94, "0 Power [dBm]"=w93, "Time"=w95, "1 Freq. [MHz]"="10", "1 Power [dBm]"="-80") -> (w104:T17)
      }
      n38 = Bundle By Name(cluster=w83, "2 Freq. [MHz]"=w78, "2 Power [dBm]"=w77, "3 Freq. [MHz]"=w78, "3 Power [dBm]"=w77, "Serial Port"=refnum<visa-resource-name> "COM1", "Ramp Channels"=w82) -> (w81:T15)
      n39 = Build Array(w81) -> (w80:T14)
    }
    frame #4 {
      n40 = Unbundle By Name(w112) -> ("SRS Ramps"=w110:T19)
      n41 = Index Array(array=w110, index=0) -> (element=w108:T20)
      n42 = for {
        tunnel: w111 -> [w122] mode=indexing
        tunnel: w108 -> [w117]
        tunnel: [w119] -> w107 mode=indexing
        n43 = Unbundle By Name(w122) -> ("Output"=w121:cluster{"Time Values":dbl[], dbl[]}[], "SRS Selection"=w120:T21, "lattice ramp"=w118:T22)
        n44 = Unbundle By Name(w117) -> ("lattice ramp"=w116:cluster{"dt":string, "formula":string}[])
        n45 = Index Array(array=w116, index=0) -> (element=w114:cluster{"dt":string, "formula":string})
        n46 = for {
          tunnel: w118 -> [w133] mode=indexing
          tunnel: w114 -> [w128]
          tunnel: [w127] -> w113 mode=indexing
          n47 = Unbundle By Name(w133) -> ("dt"=w124:dbl, "a"=w131:dbl, "b"=w130:dbl, "c"=w129:dbl, "Ramp Type"=w132:T23)
          n48 = case shown="\"HGauss (a to b, width c)\"" w132 {
            tunnel: w131 -> [w135 w139 w144 w149 w153 w158]
            tunnel: w130 -> [_ w137 w142 w147 w151 w156]
            tunnel: w129 -> [_ _ w141 w146 _ w155]
            tunnel: [w134 w138 w143 w148 w152 w157] -> w123
            frame "Hold=a", Default {
              n49 = Format Into String(format string="%.3f", w135) -> (resulting string=w134:string)  [unwired: 2 in, 1 out]
            }
            frame "Lin (a to b)" {
              n50 = Format Into String(format string="LineRamp(f, %.3f, %.3f)", w139, w137) -> (resulting string=w138:string)  [unwired: 2 in, 1 out]
            }
            frame "Exp, (a to b with tau=c)" {
              n51 = Format Into String(format string="ExpRamp(t, %.3f, %.3f,%.3f)", w144, w142, w141) -> (resulting string=w143:string)  [unwired: 2 in, 1 out]
            }
            frame "Sin=a+b*sin(2*pi*c*t)" {
              n52 = Format Into String(format string="SinRamp(t, %.3f, %.3f,%.3f)", w149, w147, w146) -> (resulting string=w148:string)  [unwired: 2 in, 1 out]
            }
            frame "Blackman (a = amp)" {
              n53 = Format Into String(format string="Blackman(f, %.3f, %.3f)", w153, w151) -> (resulting string=w152:string)  [unwired: 2 in, 1 out]
            }
            frame "HGauss (a to b, width c)" {
              n54 = Format Into String(format string="HalfGaussRamp(t, %.3f, %.3f,%.3f)", w158, w156, w155) -> (resulting string=w157:string)  [unwired: 2 in, 1 out]
            }
          }
          n55 = Format Into String(format string="%.4e", w124) -> (resulting string=w125:string)  [unwired: 2 in, 1 out]
          n56 = Bundle By Name(cluster=w128, "dt"=w125, "formula"=w123) -> (w127:cluster{"dt":string, "formula":string})
        }
        n57 = Bundle By Name(cluster=w117, "Output"=w121, "SRS Selection"=w120, "lattice ramp"=w113) -> (w119:T20)
      }
    }
    frame #5 {
      # "Master AO Ramp List"
      n58 = Unbundle By Name(w165) -> ("Master AO Ramp List"=w164:T24)
      n59 = Index Array(array=w164, index=0) -> (element=w162:T25)
      n60 = for {
        tunnel: w162 -> [w179]
        tunnel: w161 -> [w178] mode=indexing
        tunnel: [w173] -> w160 mode=indexing
        n61 = Unbundle By Name(w178) -> ("Ramp time"=w168:dbl, "Nsteps"=w167:u32, "Ramp index"=w177:u32, "Start Values"=w176:dbl[], "Stop Values"=w175:dbl[])
        n62 = for {
          tunnel: w176 -> [w181] mode=indexing
          tunnel: w175 -> [w180] mode=indexing
          tunnel: [w182] -> w174 mode=indexing
          n63 = Format Into String(format string=" LineRamp(f, %.3f, %.3f)", w181, w180) -> (resulting string=w182:string)  [unwired: 2 in, 1 out]
        }
        n64 = Max & Min(x=1, y=w167) -> (max(x,y)=w172:u32)  [unwired: 1 out]
        n65 = Divide(x=w168, y=w172) -> (x/y=w170:dbl)
        n66 = Format Into String(format string="%.3e", w168) -> (resulting string=w169:string)  [unwired: 2 in, 1 out]
        n67 = Bundle By Name(cluster=w179, "Ramp time [s]"=w169, "Step size [s]"=w170, "Ramp index"=w177, "Ramp Array"=w174) -> (w173:T25)
      }
    }
    frame #6 {
      # "This needs to be reverse\nordered.  The sort works\nbecause the \"first\" element\nof the cluster is the ramp index."
      # "Master AO Staging List"
      n68 = Unbundle By Name(w194) -> ("Master AO Ramp List"=w193:T24)
      n69 = Index Array(array=w193, index=0) -> (element=w191:T25)
      n70 = for {
        tunnel: w191 -> [w197]
        tunnel: w190 -> [w206] mode=indexing
        shift-right: [w201] -> w186
        shift-left: w189 -> [w202]
        tunnel: w187 -> [w199]
        shift-right: [w198] -> _
        shift-left: 0 -> [w200]
        i -> [w195]
        n71 = Unbundle By Name(w206) -> ("Delay (s)"=w196:dbl, "Output Bits"=w205:bool[])
        n72 = Index Array(array=w205, index=23) -> (element=w203:bool)
        n73 = case shown="True" w203 {
          tunnel: w202 -> [w208 w212]
          tunnel: [w208 w210] -> w201
          tunnel: w200 -> [w207 w214]
          tunnel: w199 -> [_ w219]
          tunnel: [w207 w220] -> w198
          tunnel: w197 -> [_ w221]
          tunnel: w196 -> [_ w216]
          tunnel: w195 -> [_ w209]
          frame False {
          }
          frame True {
            n74 = Index Array(array=w219, index (row)=w214) -> (element=w218:dbl[])  [unwired: 1 in]
            n75 = for {
              tunnel: [w224] -> w213 mode=indexing
              tunnel: w218 -> [w222] mode=indexing
              n76 = Format Into String(format string="%.3f", w222) -> (resulting string=w224:string)  [unwired: 2 in, 1 out]
            }
            n77 = Format Into String(format string="%.3e", w216) -> (resulting string=w215:string)  [unwired: 2 in, 1 out]
            n78 = Bundle By Name(cluster=w221, "Ramp time [s]"=w215, "Step size [s]"=w216, "Ramp index"=w209, "Ramp Array"=w213) -> (w211:T25)
            n79 = Insert Into Array(array=w212, new element=w211) -> (w210:T24)  [unwired: 1 in]
            n80 = Increment(x=w214) -> (x+1=w220:i32)
          }
        }
      }
      n81 = Sort 1D Array(array=w186) -> (sorted array=w185:T24)
      n82 = Reverse 1D Array(array=w185) -> (reversed array=w184:T24)
    }
    frame #7 {
      # "Slave AO Ramp List"
      n83 = Unbundle By Name(w230) -> ("Slave AO Ramp List"=w229:T24)
      n84 = Index Array(array=w229, index=0) -> (element=w227:T25)
      n85 = for {
        tunnel: w227 -> [w244]
        tunnel: w226 -> [w243] mode=indexing
        tunnel: [w238] -> w225 mode=indexing
        n86 = Unbundle By Name(w243) -> ("Ramp time"=w234:dbl, "Nsteps"=w236:u32, "Ramp index"=w242:u32, "Start Values"=w241:dbl[], "Stop Values"=w240:dbl[])
        n87 = for {
          tunnel: w241 -> [w246] mode=indexing
          tunnel: w240 -> [w245] mode=indexing
          tunnel: [w248] -> w239 mode=indexing
          n88 = Format Into String(format string=" LineRamp(f, %.3f, %.3f)", w246, w245) -> (resulting string=w248:string)  [unwired: 2 in, 1 out]
        }
        n89 = Max & Min(x=1, y=w236) -> (max(x,y)=w233:u32)  [unwired: 1 out]
        n90 = Divide(x=w234, y=w233) -> (x/y=w232:dbl)
        n91 = Format Into String(format string="%.3e", w234) -> (resulting string=w237:string)  [unwired: 2 in, 1 out]
        n92 = Bundle By Name(cluster=w244, "Ramp time [s]"=w237, "Step size [s]"=w232, "Ramp index"=w242, "Ramp Array"=w239) -> (w238:T25)
      }
    }
    frame #8 {
      # "This needs to be reverse\nordered.  The sort works\nbecause the \"first\" element\nof the cluster is the ramp index."
      # "Slave AO Staging List"
      n93 = Unbundle By Name(w259) -> ("Master AO Ramp List"=w258:T24)
      n94 = Index Array(array=w258, index=0) -> (element=w256:T25)
      n95 = for {
        tunnel: w256 -> [w262]
        tunnel: w250 -> [w271] mode=indexing
        shift-right: [w266] -> w254
        shift-left: w249 -> [w267]
        tunnel: w251 -> [w264]
        shift-right: [w263] -> _
        shift-left: 0 -> [w265]
        i -> [w260]
        n96 = Unbundle By Name(w271) -> ("Delay (s)"=w261:dbl, "Output Bits"=w270:bool[])
        n97 = Index Array(array=w270, index=23) -> (element=w268:bool)
        n98 = case shown="True" w268 {
          tunnel: w267 -> [w273 w277]
          tunnel: [w273 w275] -> w266
          tunnel: w265 -> [w272 w279]
          tunnel: w264 -> [_ w284]
          tunnel: [w272 w285] -> w263
          tunnel: w262 -> [_ w286]
          tunnel: w261 -> [_ w281]
          tunnel: w260 -> [_ w274]
          frame False {
          }
          frame True {
            n99 = Index Array(array=w284, index (row)=w279) -> (element=w283:dbl[])  [unwired: 1 in]
            n100 = for {
              tunnel: [w289] -> w278 mode=indexing
              tunnel: w283 -> [w287] mode=indexing
              n101 = Format Into String(format string="%.3f", w287) -> (resulting string=w289:string)  [unwired: 2 in, 1 out]
            }
            n102 = Format Into String(format string="%.3e", w281) -> (resulting string=w280:string)  [unwired: 2 in, 1 out]
            n103 = Bundle By Name(cluster=w286, "Ramp time [s]"=w280, "Step size [s]"=w281, "Ramp index"=w274, "Ramp Array"=w278) -> (w276:T25)
            n104 = Insert Into Array(array=w277, new element=w276) -> (w275:T24)  [unwired: 1 in]
            n105 = Increment(x=w279) -> (x+1=w285:i32)
          }
        }
      }
      n106 = Sort 1D Array(array=w254) -> (sorted array=w253:T24)
      n107 = Reverse 1D Array(array=w253) -> (reversed array=w252:T24)
    }
  }
  n108 = Bundle By Name(cluster=w1, "Master PB Staging List"=w13, "Master AO Ramp List"=w9, "Slave PB Staging List"=w12, "Slave AO Ramp List"=w8, "Novatech Ramps"=w7, "Sequencing Info"=w11, "SRS Ramps"=w10, "Master Novatech Ramp List"=w2) -> (→"Paramaters":T1)
